vi "9219_Update Channels.vi"(8 "error in (no error)":errorcluster, 10 "9219 In":refnum<class "9219.lvclass">, 11 "Node Ptr In":T1 format="%.0x") -> (0 "error out":errorcluster, 2 "9219 Out":refnum<class "9219.lvclass">, 3 "Node Ptr Out":T1 format="%.0x")   [LabVIEW 2011, in "Modules.lvlib" / "9219.lvclass"]
uses:
  9219.lvclass
  <vilib>/NI Veristand/Custom Device API/Custom Device Item Ref.ctl
  9219.lvclass/9219.ctl
  <vilib>/NI Veristand/Custom Device API/Custom Device API.lvlib
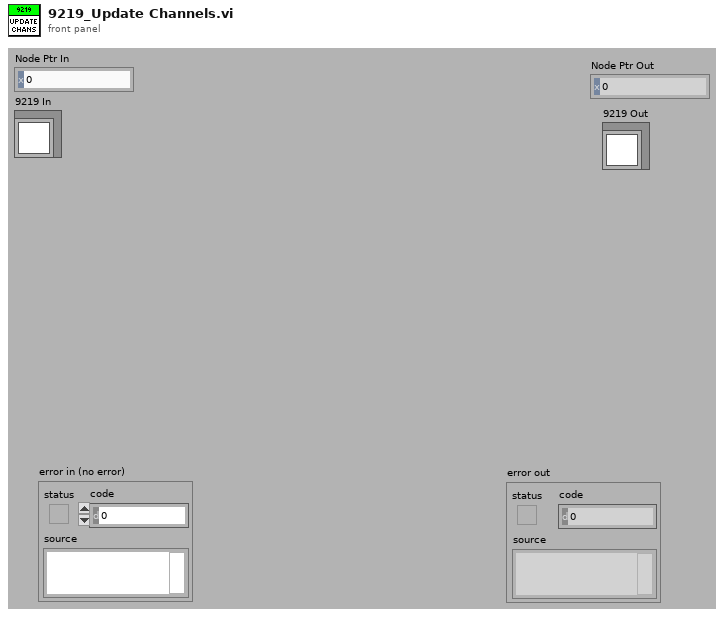
[diagram p1: front panel]
types:
  T1 = typedef "Custom Device API.lvlib/Custom Device Item Ref.ctl" = u64
  T2 = cluster{"Degree range":u32, "Digital threshold":dbl, "Range / Mode":u32, "RTD type":u32, "RTD A":dbl, "RTD B":dbl, "RTD C":dbl, "RTD Ro":dbl, "Thermocouple type":u32}[]
  T3 = typedef "Custom Device API.lvlib/Custom Device Channel.ctl" = cluster{"Type":T4, "Units":string, "Default Value":dbl, "Faultable":bool, "Scalable":bool}
  T4 = typedef "Custom Device API.lvlib/Custom Device Channel Type.ctl" = enum16{"Input", "Output"}
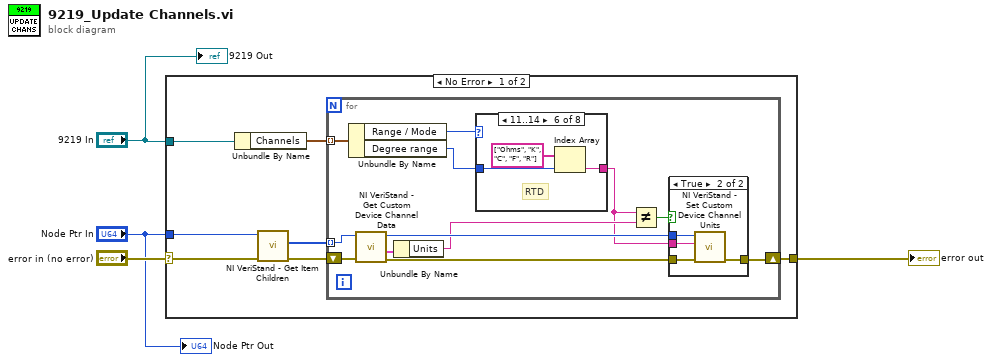
[diagram p0: block diagram]
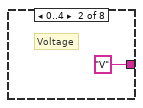
[diagram p3: hidden frame]
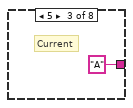
[diagram p4: hidden frame]
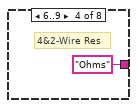
[diagram p5: hidden frame]
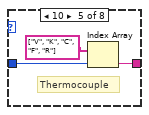
[diagram p6: hidden frame]
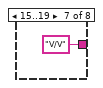
[diagram p7: hidden frame]
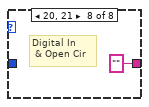
[diagram p8: hidden frame]
diagram:
  n1 = case shown="No Error" "error in (no error)" {
    selector: "error in (no error)" -> [w11 w40]
    tunnel: [w5 w40] -> w3
    tunnel: "Node Ptr In" -> [w10 _]
    tunnel: "9219 In" -> [w9 _]
    frame No Error {
      n2 = Unbundle By Name(w9) -> ("Channels"=w6:T2)
      n3 = call <vilib>:"NI VeriStand - Get Item Children.vi"("error in (no error)"=w11, "Item Ref in"=w10) -> ("error out"=w8:errorcluster, "Child Refs"=w7:T1[])  [unwired: 6 in, 2 out]
      n4 = for {
        shift-right: [w23] -> w5
        shift-left: w8 -> [w22]
        tunnel: w7 -> [w21] mode=indexing
        tunnel: w6 -> [w15] mode=indexing
        n5 = Unbundle By Name(w15) -> ("Range / Mode"=w14:u32, "Degree range"=w12:u32)
        n6 = call <vilib>:"NI VeriStand - Get Custom Device Channel Data.vi"("error in (no error)"=w22, "Channel Ref in"=w21) -> ("error out"=w19:errorcluster, "Channel"=w20:T3, "Channel Ref out"=w18:T1)  [unwired: 4 in, 3 out]
        n7 = Unbundle By Name(w20) -> ("Units"=w16:string)
        n8 = case shown="11..14" w14 {
          tunnel: [_ "V" "A" "Ohms" w28 w32 "V/V" ""] -> w13
          tunnel: w12 -> [_ _ _ _ w27 w31 _ _]
          frame Default {
          }
          frame 0..4 {
            # "Voltage"
          }
          frame 5 {
            # "Current"
          }
          frame 6..9 {
            # "4&2-Wire Res"
          }
          frame 10 {
            # "Thermocouple"
            n9 = Index Array(array=string[] ["V", "K", "C", "F", "R"], index=w27) -> (element=w28:string)
          }
          frame 11..14 {
            # "RTD"
            n10 = Index Array(array=string[] ["Ohms", "K", "C", "F", "R"], index=w31) -> (element=w32:string)
          }
          frame 15..19 {
          }
          frame 20, 21 {
            # "Digital In\n & Open Cir"
          }
        }
        n11 = Not Equal?(x=w13, y=w16) -> (x != y?=w17:bool)
        n12 = case shown="True" w17 {
          tunnel: w18 -> [_ w39]
          tunnel: w13 -> [_ w38]
          tunnel: w19 -> [w35 w37]
          tunnel: [w35 w36] -> w23
          frame False {
          }
          frame True {
            n13 = call <vilib>:"NI VeriStand - Set Custom Device Channel Units.vi"("error in (no error)"=w37, "Units"=w38, "Channel Ref in"=w39) -> ("error out"=w36:errorcluster)  [unwired: 7 in, 1 out]
          }
        }
      }
    }
    frame Error {
    }
  }
  "error out" <- w3
  "9219 Out" <- "9219 In"
  "Node Ptr Out" <- "Node Ptr In"
